vi "InitCamera.vi"(7 "Up Direction":T1={"X"=0.0, "Y"=1.0, "Z"=0.0}, 8 "error in (no error)":errorcluster, 9 "Target":T1, 10 "Camera Position":T1={"X"=0.0, "Y"=0.0, "Z"=5.0}, 11 "3D Scene in":refnum<class "3D Scene.lvclass">) -> (0 "error out":errorcluster, 3 "3D Scene out":refnum<class "3D Scene.lvclass">)   [LabVIEW 2015, in "3D Scene.lvclass"]
uses:
  3D Scene.lvclass
  <vilib>/Utility/miscctls.llb/LV3DPointTypeDef.ctl
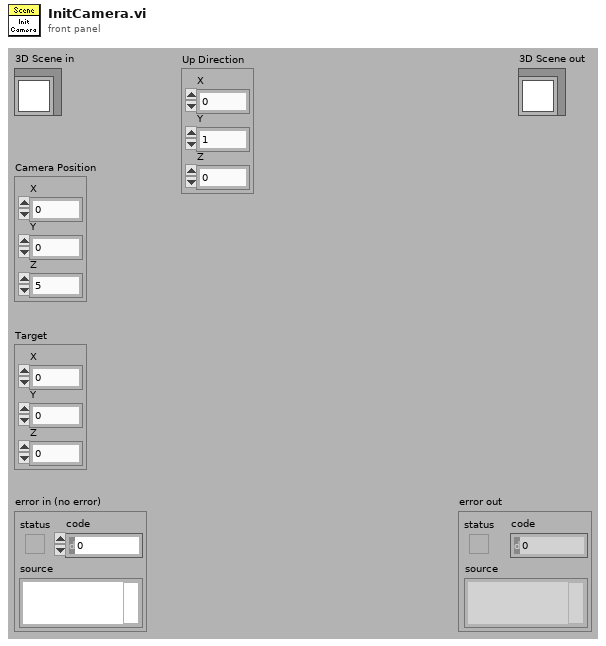
[diagram p1: front panel]
types:
  T1 = typedef "LV3DPointTypeDef.ctl" = cluster{"X":sgl, "Y":sgl, "Z":sgl}
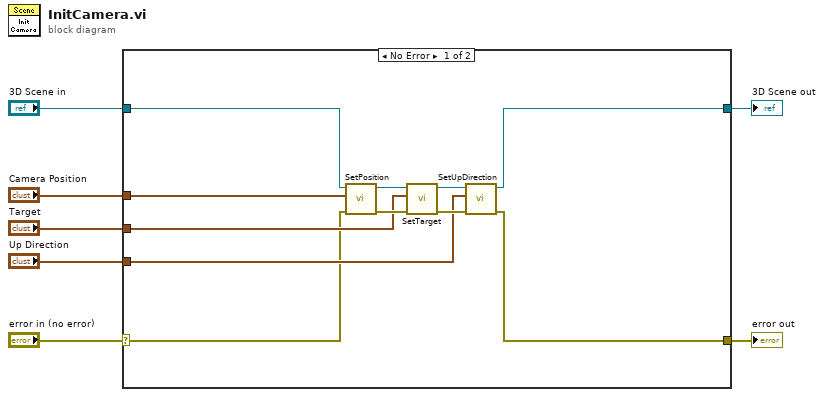
[diagram p0: block diagram]
diagram:
  n1 = case shown="No Error" "error in (no error)" {
    selector: "error in (no error)" -> [w8 w20]
    tunnel: [w10 w20] -> w6
    tunnel: [w9 w19] -> w4
    tunnel: "3D Scene in" -> [w18 w19]
    tunnel: "Camera Position" -> [w17 _]
    tunnel: "Target" -> [w12 _]
    tunnel: "Up Direction" -> [w11 _]
    frame No Error {
      n2 = call "SetPosition.vi"("error in (no error)"=w8, "Position"=w17, "3D Scene in"=w18) -> ("error out"=w14:errorcluster, "3D Scene out"=w16:refnum<class "3D Scene.lvclass">)  [unwired: 7 in]
      n3 = call "SetTarget.vi"("error in (no error)"=w14, "Target"=w12, "3D Scene in"=w16) -> ("error out"=w13:errorcluster, "3D Scene out"=w15:refnum<class "3D Scene.lvclass">)  [unwired: 7 in]
      n4 = call "SetUpDirection.vi"("error in (no error)"=w13, "Up Direction"=w11, "3D Scene in"=w15) -> ("error out"=w10:errorcluster, "3D Scene out"=w9:refnum<class "3D Scene.lvclass">)  [unwired: 7 in]
    }
    frame Error {
    }
  }
  "error out" <- w6
  "3D Scene out" <- w4
